vi "Write Input Registers.vi"(8 "error in (no error)":errorcluster, 9 "register values":u16[](array[numeric]), 10 "starting address":u16, 11 "Device Data Model in":refnum<class "Device Data Model.lvclass">) -> (0 "error out":errorcluster, 3 "Device Data Model out":refnum<class "Device Data Model.lvclass">)   [LabVIEW 2014, in "MyLib.lvlib" / "Device Data Model.lvclass"]
doc: "Writes the values of multiple input register values in series, starting at address M."
uses:
  Device Data Model.lvclass
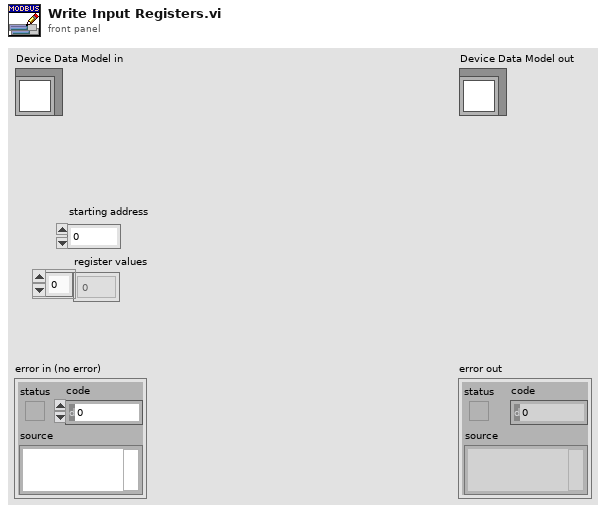
[diagram p1: front panel]
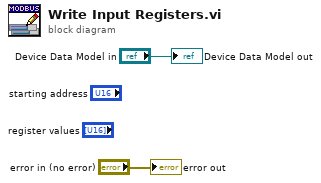
[diagram p0: block diagram]
diagram:
  "error out" <- "error in (no error)"
  "Device Data Model out" <- "Device Data Model in"
